vi "Write path.vi"(8 "error in (no error)":errorcluster, 10 "path":string, 11 "URI in":refnum<class "URI.lvclass">) -> (0 "error out":errorcluster, 3 "URI out":refnum<class "URI.lvclass">)   [LabVIEW 2013, in "openURI.lvlib" / "URI.lvclass"]
uses:
  URI.lvclass
  URI.lvclass/URI.ctl
  components/path/URI-Component.Path.lvclass
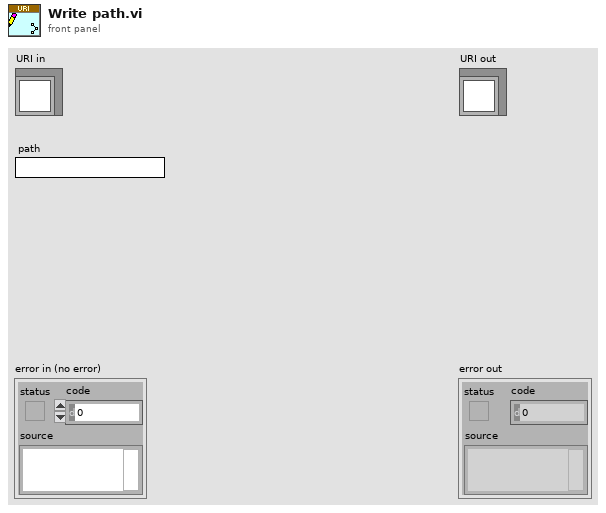
[diagram p1: front panel]
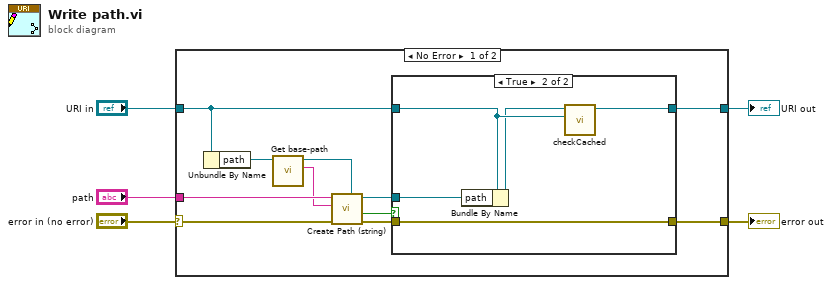
[diagram p0: block diagram]
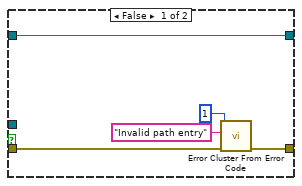
[diagram p2: hidden frame]
diagram:
  n1 = case shown="No Error" "error in (no error)" {
    selector: "error in (no error)" -> [w13 w27]
    tunnel: [w10 w27] -> w4
    tunnel: [w16 w28] -> w2
    tunnel: "URI in" -> [w9 w28]
    tunnel: "path" -> [w15 _]
    frame No Error {
      n2 = Unbundle By Name(w9) -> ("path"=w8:refnum<class "URI-Component.Path.lvclass">)
      n3 = call "Get base-path.vi"("URI-Component.Path in"=w8) -> ("base-path"=w6:string, "URI-Component.Path out"=w7:refnum<class "URI-Component.Path.lvclass">)  [unwired: 8 in, 1 out]
      n4 = call "Create Path (string).vi"("URI-Component.Path"=w7, "error in (no error)"=w13, "base-path"=w6, "Path"=w15) -> ("error out"=w11:errorcluster, "Valid"=w12:bool, "URI-Component.Path"=w14:refnum<class "URI-Component.Path.lvclass">)  [unwired: 4 in, 1 out]
      n5 = case shown="True" w12 {
        tunnel: w9 -> [w21 w26]
        tunnel: [w21 w24] -> w16
        tunnel: w14 -> [_ w23]
        tunnel: w11 -> [w19 w22]
        tunnel: [w20 w22] -> w10
        frame False {
          n6 = call <vilib>:"Error Cluster From Error Code.vi"("error in (no error)"=w19, "error message (\"\")"="Invalid path entry" ("error message (\"\")"), "error code (0)"=1) -> ("error out"=w20:errorcluster)  [unwired: 6 in]
        }
        frame True {
          n7 = Bundle By Name(cluster=w26, "path"=w23) -> (w25:refnum<class "URI.lvclass">)
          n8 = call "checkCached.vi"("Old"=w26, "New URI"=w25) -> ("URI"=w24:refnum<class "URI.lvclass">)  [unwired: 9 in]
        }
      }
    }
    frame Error {
    }
  }
  "error out" <- w4
  "URI out" <- w2
